vi "Main_Add User.vi"(8 "error in (no error)":errorcluster caption="에러 입력(에러 없음)") -> (0 "error out":errorcluster caption="에러 출력")   [LabVIEW 2019]
uses:
  <vilib>/Utility/config.llb/Read Key (String).vi
  <vilib>/Utility/config.llb/Read Key (U32).vi
  <vilib>/Utility/config.llb/Write Key (String).vi
  <vilib>/Utility/config.llb/Write Key (I32).vi
  <vilib>/Utility/config.llb/NI_LVConfig.lvlib
panel:
  out "권한":u32[](array[numeric])
  out "PW 2":string[](array[string])
  out "ID 2":string[](array[string])
  out "추가된 배열":string[][](array[string])
  in  "exit":bool
  in  "리스트":i32[](listbox) caption="User List"
  in  "제거 버튼":bool
  in  "추가 버튼":bool
  in  "PW":string="품명"
  in  "열거형":enum16{"Administrator", "Operator"}(ring) caption="User Authority"
  in  "ID":string="품명"
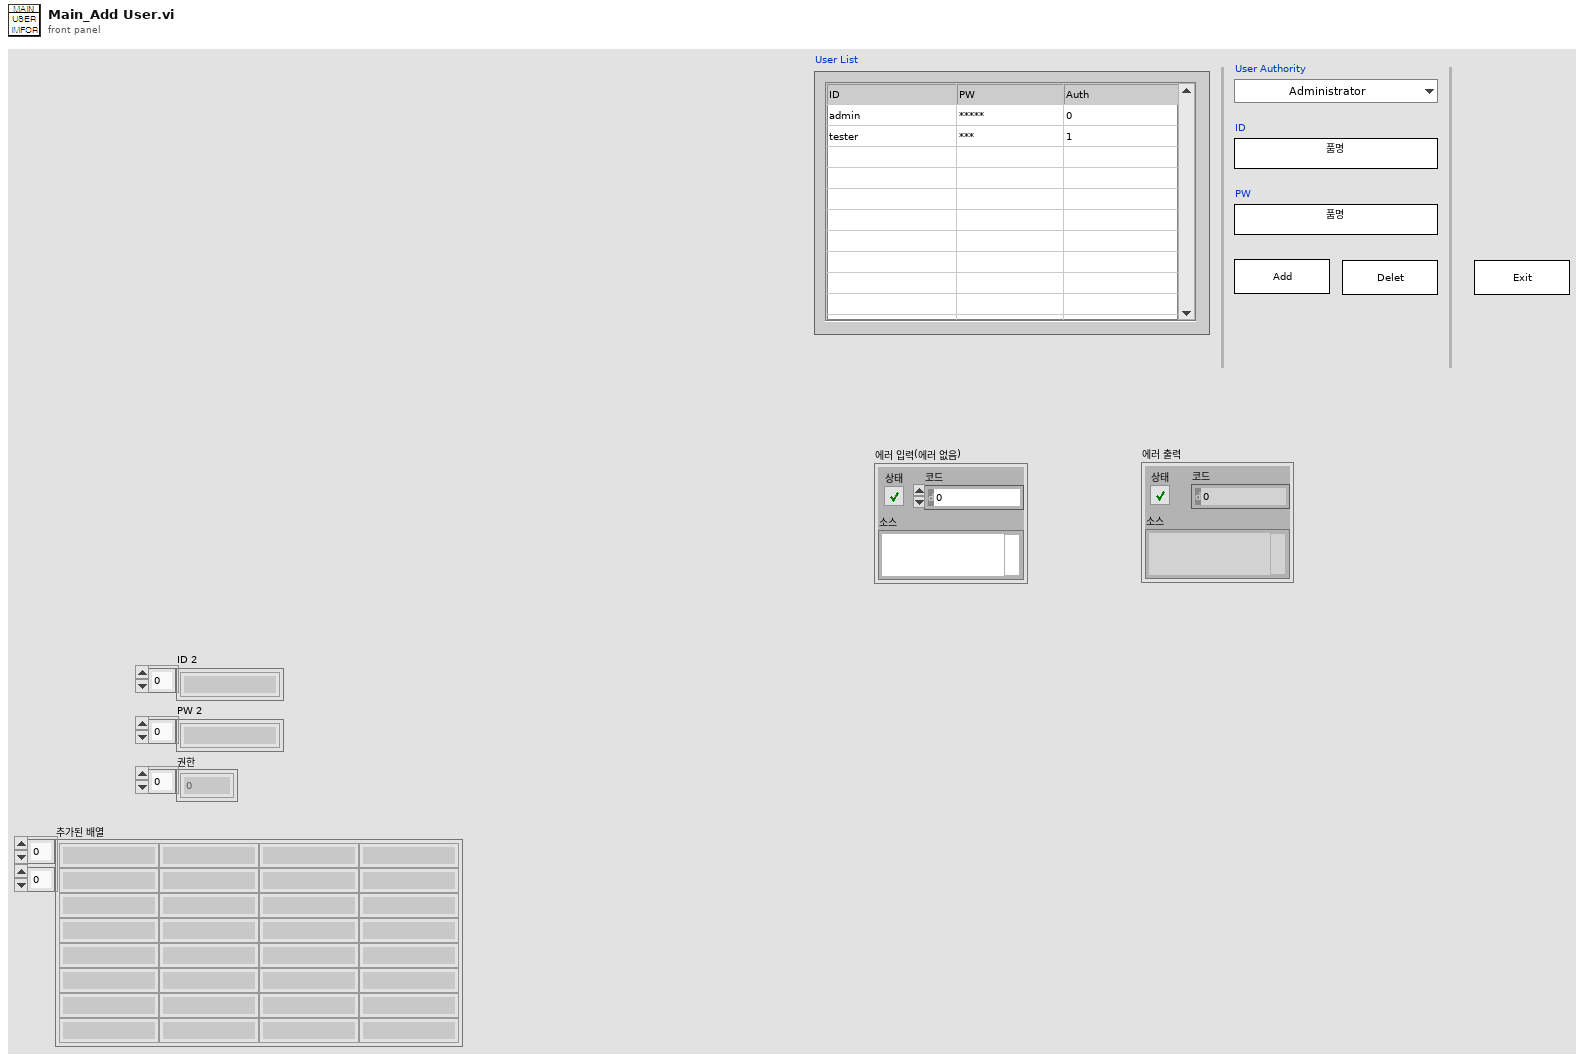
[diagram p1: front panel]
types:
  T1 = typedef "NI_LVConfig.lvlib/Config Data RefNum.ctl" = refnum<k1>
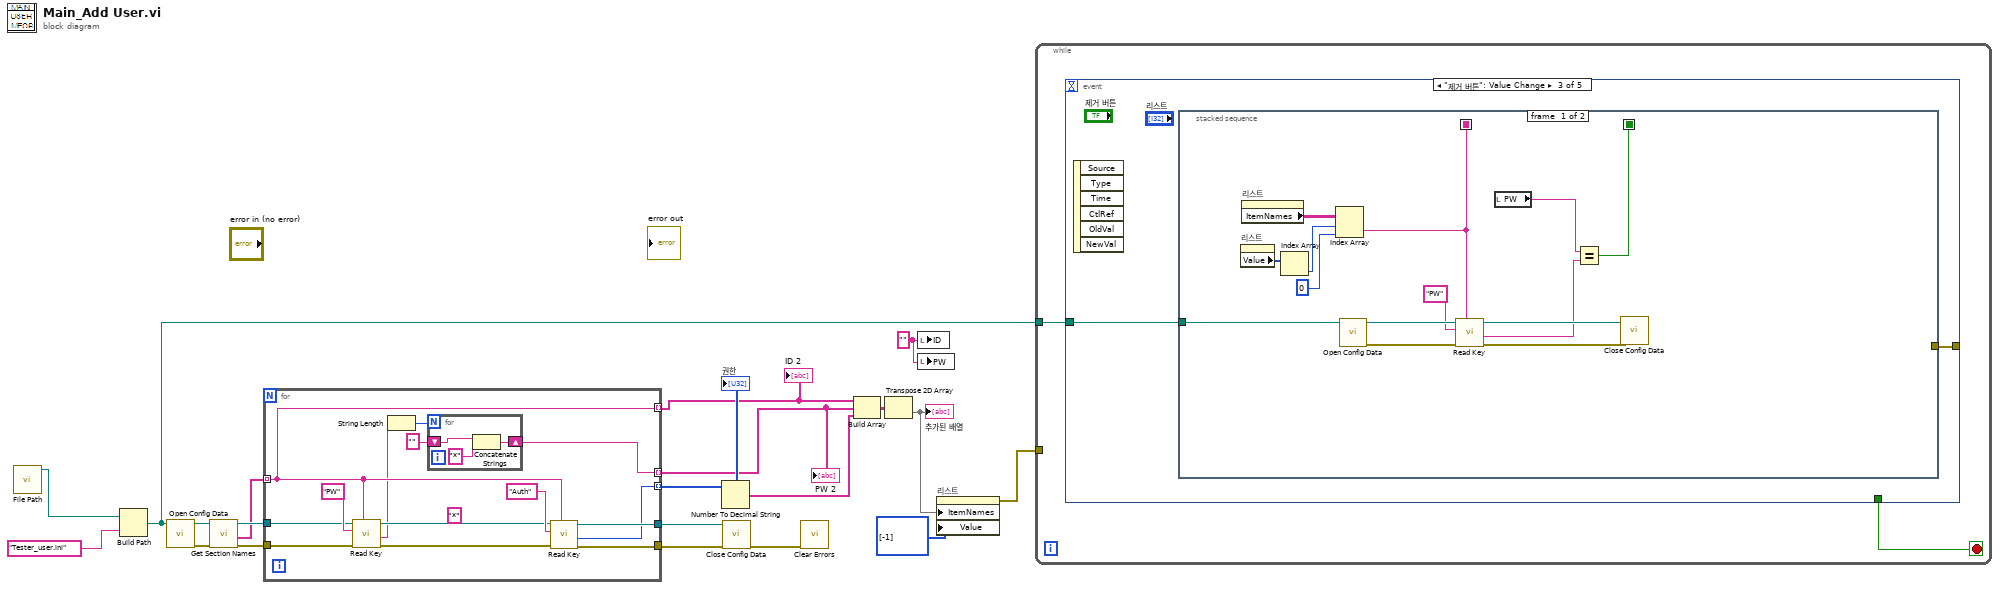
[diagram p0: block diagram]
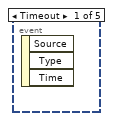
[diagram p2: hidden frame]
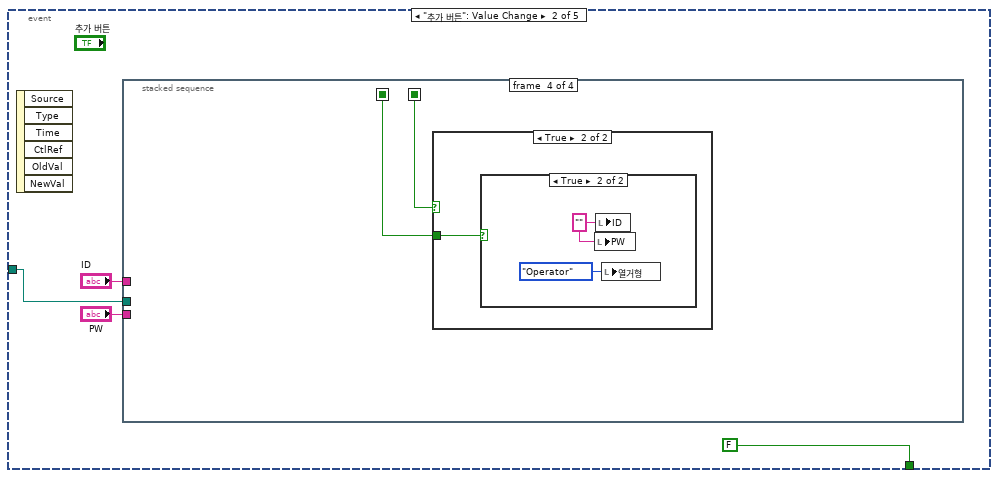
[diagram p3: hidden frame]
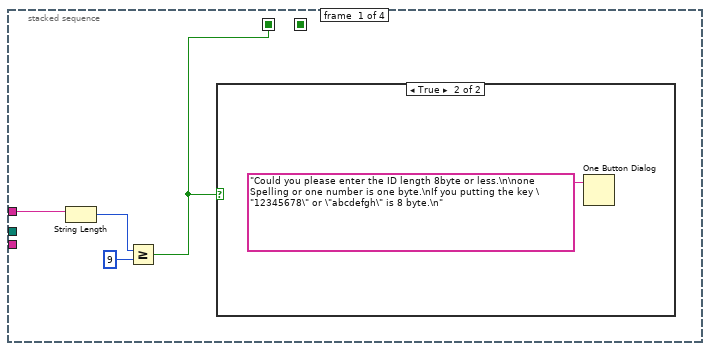
[diagram p4: hidden frame]
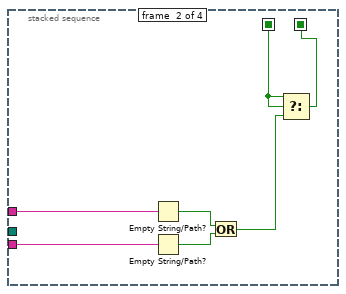
[diagram p6: hidden frame]
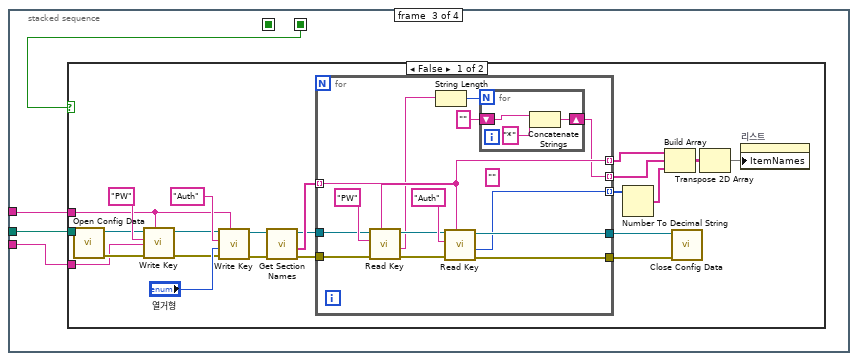
[diagram p7: hidden frame]
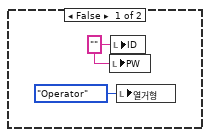
[diagram p9: hidden frame]
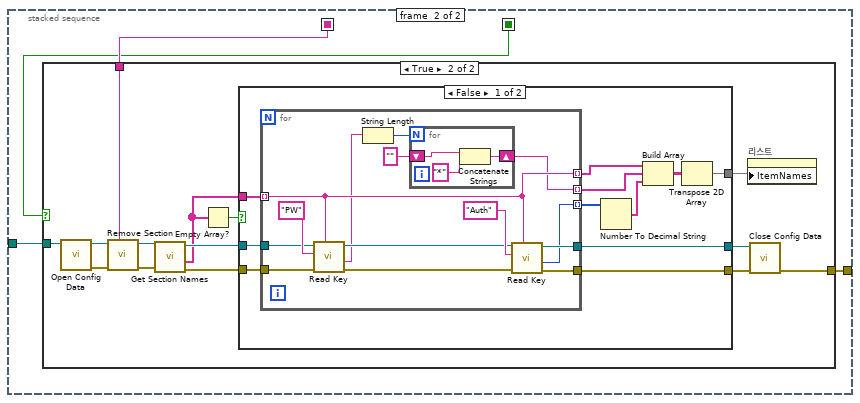
[diagram p11: hidden frame]
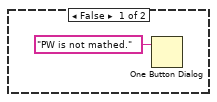
[diagram p12: hidden frame]
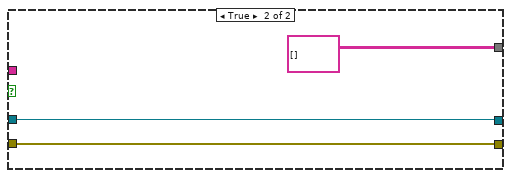
[diagram p13: hidden frame]
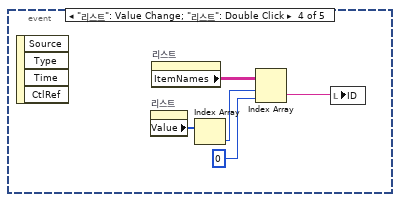
[diagram p14: hidden frame]
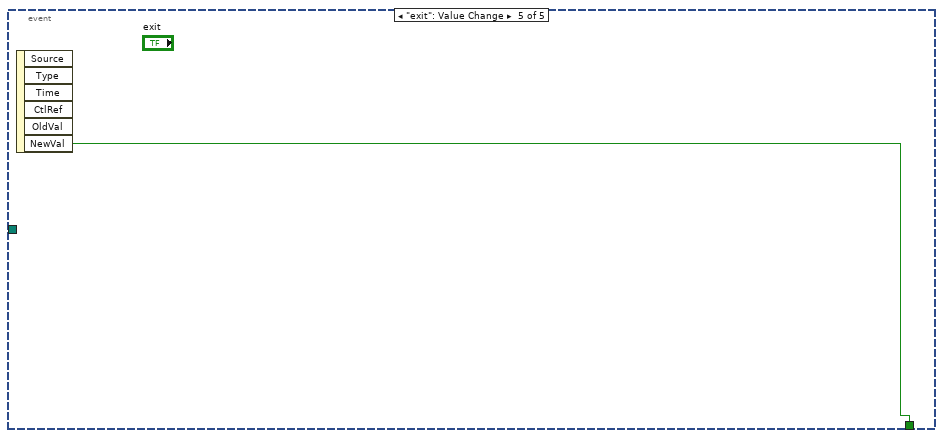
[diagram p15: hidden frame]
diagram:
  w4 = "" ("ID")
  n1 = call "File Path.vi"() -> ("condition"=w1:path)  [unwired: 7 in, 4 out]
  n2 = Build Path(base path=w1, name or relative path="Tester_user.ini" ("이름 또는 상대 경로")) -> (appended path=w6:path)
  n3 = call <vilib>:"Open Config Data.vi"("configuration file path"=w6) -> ("error out"=w15:errorcluster, "refnum"=w17:T1)  [unwired: 8 in, 1 out]
  n4 = call <vilib>:"Get Section Names.vi"("error in (no error)"=w15, "refnum"=w17) -> ("error out"=w14:errorcluster, "section names"=w13:string[], "refnum out"=w16:T1)  [unwired: 7 in]
  n5 = for {
    tunnel: [w34] -> w19
    tunnel: [w33] -> w18
    tunnel: w16 -> [w28]
    tunnel: w14 -> [w27]
    tunnel: w13 -> [w26] mode=indexing
    tunnel: [w26] -> w11 mode=indexing
    tunnel: [w22] -> w10 mode=indexing
    tunnel: [w25] -> w12 mode=indexing
    (unwired) "*"
    n6 = call-poly <vilib>:"Read Key.vi"("section"=w26, "error in (no error)"=w27, "key"="PW", "refnum"=w28) -> ("error out"=w30:errorcluster, "value"=w24:string, "refnum out"=w29:T1)  [unwired: 4 in, 1 out]
    n7 = String Length(string=w24) -> (length=w23:i32)
    n8 = for {
      N: w23 -> [_]
      shift-right: [w36] -> w22
      shift-left: "" -> [w35]
      n9 = Concatenate Strings(w35, "*") -> (w36:string)
    }
    n10 = call-poly <vilib>:"Read Key.vi"("section"=w26, "error in (no error)"=w30, "key"="Auth" ("default value"), "refnum"=w29) -> ("error out"=w34:errorcluster, "value"=w25:u32, "refnum out"=w33:T1)  [unwired: 4 in, 1 out]
  }
  "ID 2" <- w11
  "PW 2" <- w10
  "권한" <- w12
  n11 = Number To Decimal String(number=w12) -> (decimal integer string=w9:string[])  [unwired: 1 in]
  n12 = call <vilib>:"Close Config Data.vi"("error in (no error)"=w19, "refnum"=w18) -> ("error out"=w3:errorcluster)  [unwired: 8 in, 1 out]
  n13 = call <vilib>:"Clear Errors.vi"("error in (no error)"=w3) -> ()  [unwired: 5 in, 2 out]
  n14 = Build Array(w11, w10, w9) -> (w8:string[][])
  n15 = Transpose 2D Array(2D array=w8) -> (transposed array=w7:string[][])
  "추가된 배열" <- w7
  n16 = local write "ID"(w4) -> ()
  n17 = local write "PW"(w4) -> ()
  n18 = property on="리스트" class="MCListbox (strict)"("ItemNames"=w7, "Value"=i32[] [-1] ("리스트")) -> (error out=w5:errorcluster)  [unwired: 2 in, 1 out]
  n19 = while {
    tunnel: w6 -> [w39]
    tunnel: w5 -> [_]
    stop <- w38 stop-if-true
    n20 = event shown="[2] \"제거 버튼\": Value Change" {
      selector: _ -> [_ _ _ _ _]
      dyn-events: _ -> [_ _ _ _ _]
      timeout: _ -> [_ _ _ _ _]
      tunnel: w39 -> [_ w43 w108 _ _]
      tunnel: [_ FALSE _ _ w178] -> w38
      tunnel: [_ _ w107 _ _] -> _
      event Timeout {
        n21 = event-data() -> ()  [unwired: 1 in, 3 out]
      }
      event "추가 버튼": Value Change {
        n22 = event-data() -> ()  [unwired: 1 in, 6 out]
        n23 = stacked-sequence {
          seq-local: [_ w49 _ _] -> [_ _ w56 w101]
          seq-local: [w44 _ _ _] -> [_ w51 _ w100]
          tunnel: w43 -> [_ _ w59 _]
          tunnel: "ID" -> [w45 w53 w58 _]
          tunnel: "PW" -> [_ w52 w57 _]
          frame #0 {
            n24 = String Length(string=w45) -> (length=w47:i32)
            n25 = Greater Or Equal?(x=w47, y=9) -> (x >= y?=w44:bool)
            n26 = case shown="True" w44 {
              frame False {
              }
              frame True {
                n27 = One Button Dialog(message="Could you please enter the ID length 8byte or less.\n\none Spelling or one number is one byte.\nIf you putting the key \"12345678\" or \"abcdefgh\" is 8 byte.\n" ("메시지")) -> ()  [unwired: 1 in, 1 out]
              }
            }
          }
          frame #1 {
            n28 = Empty String/Path?(string/path=w53) -> (empty?=w55:bool)
            n29 = Empty String/Path?(string/path=w52) -> (empty?=w54:bool)
            n30 = Or(x=w55, y=w54) -> (x .or. y?=w50:bool)
            n31 = Select(t=w51, s=w51, f=w50) -> (s? t:f=w49:bool)
          }
          frame #2 {
            n32 = case shown="False" w56 {
              tunnel: w59 -> [w75 _]
              tunnel: w58 -> [w61 _]
              tunnel: w57 -> [w60 _]
              frame False {
                n33 = call <vilib>:"Open Config Data.vi"("configuration file path"=w75) -> ("error out"=w77:errorcluster, "refnum"=w76:T1)  [unwired: 8 in, 1 out]
                n34 = call-poly <vilib>:"Write Key.vi"("section"=w61, "error in (no error)"=w77, "value"=w60, "key"="PW", "refnum"=w76) -> ("error out"=w79:errorcluster, "refnum out"=w78:T1)  [unwired: 4 in, 1 out]
                n35 = call-poly <vilib>:"Write Key.vi"("section"=w61, "error in (no error)"=w79, "value"="열거형", "key"="Auth" ("default value"), "refnum"=w78) -> ("error out"=w62:errorcluster, "refnum out"=w63:T1)  [unwired: 4 in, 1 out]
                n36 = call <vilib>:"Get Section Names.vi"("error in (no error)"=w62, "refnum"=w63) -> ("error out"=w68:errorcluster, "section names"=w69:string[], "refnum out"=w67:T1)  [unwired: 7 in]
                n37 = for {
                  tunnel: [w96] -> w65
                  tunnel: [w95] -> w66
                  tunnel: w67 -> [w90]
                  tunnel: w68 -> [w89]
                  tunnel: w69 -> [w87] mode=indexing
                  tunnel: [w87] -> w71 mode=indexing
                  tunnel: [w83] -> w72 mode=indexing
                  tunnel: [w88] -> w70 mode=indexing
                  (unwired) "" ("value")
                  n38 = call-poly <vilib>:"Read Key.vi"("section"=w87, "error in (no error)"=w89, "key"="PW", "refnum"=w90) -> ("error out"=w92:errorcluster, "value"=w84:string, "refnum out"=w91:T1)  [unwired: 4 in, 1 out]
                  n39 = String Length(string=w84) -> (length=w86:i32)
                  n40 = call-poly <vilib>:"Read Key.vi"("section"=w87, "error in (no error)"=w92, "key"="Auth" ("default value"), "refnum"=w91) -> ("error out"=w96:errorcluster, "value"=w88:u32, "refnum out"=w95:T1)  [unwired: 4 in, 1 out]
                  n41 = for {
                    N: w86 -> [_]
                    shift-right: [w98] -> w83
                    shift-left: "" -> [w97]
                    n42 = Concatenate Strings(w97, "*") -> (w98:string)
                  }
                }
                n43 = Number To Decimal String(number=w70) -> (decimal integer string=w73:string[])  [unwired: 1 in]
                n44 = Build Array(w71, w72, w73) -> (w74:string[][])
                n45 = call <vilib>:"Close Config Data.vi"("error in (no error)"=w65, "refnum"=w66) -> ()  [unwired: 8 in, 2 out]
                n46 = Transpose 2D Array(2D array=w74) -> (transposed array=w64:string[][])
                n47 = property on="리스트" class="MCListbox (strict)"("ItemNames"=w64) -> ()  [unwired: 2 in, 2 out]
              }
              frame True {
              }
            }
          }
          frame #3 {
            n48 = case shown="True" w101 {
              tunnel: w100 -> [_ w104]
              frame False {
                w103 = "" ("ID")
                n49 = local write "PW"(w103) -> ()
                n50 = local write "ID"(w103) -> ()
                n51 = local write "열거형"(enum16{"Administrator", "Operator"}."Operator" ("열거형")) -> ()
              }
              frame True {
                n52 = case shown="True" w104 {
                  frame False {
                  }
                  frame True {
                    w105 = "" ("ID")
                    n53 = local write "PW"(w105) -> ()
                    n54 = local write "ID"(w105) -> ()
                    n55 = local write "열거형"(enum16{"Administrator", "Operator"}."Operator" ("열거형")) -> ()
                  }
                }
              }
            }
          }
        }
      }
      event "제거 버튼": Value Change {
        n56 = event-data() -> ()  [unwired: 1 in, 6 out]
        n57 = stacked-sequence {
          seq-local: [w113 _] -> [_ w124]
          seq-local: [w109 _] -> [_ w123]
          tunnel: w108 -> [w112 w126]
          tunnel: [_ w125] -> w107
          frame #0 {
            n58 = property on="리스트" class="MCListbox (strict)"() -> ("Value"=w121:i32[])  [unwired: 2 in, 2 out]
            n59 = property on="리스트" class="MCListbox (strict)"() -> ("ItemNames"=w122:string[][])  [unwired: 2 in, 2 out]
            n60 = Index Array(array=w121) -> (element=w120:i32)  [unwired: 1 in]
            n61 = Index Array(array=w122, index (row)=w120, index (col)=0 ("비활성화된 인덱스 (행)")) -> (element=w113:string)
            n62 = call <vilib>:"Open Config Data.vi"("configuration file path"=w112) -> ("error out"=w116:errorcluster, "refnum"=w115:T1)  [unwired: 8 in, 1 out]
            n63 = call-poly <vilib>:"Read Key.vi"("section"=w113, "error in (no error)"=w116, "key"="PW", "refnum"=w115) -> ("error out"=w118:errorcluster, "value"=w110:string, "refnum out"=w117:T1)  [unwired: 4 in, 1 out]
            n64 = local read "PW"() -> (w111:string)
            n65 = Equal?(x=w111, y=w110) -> (x = y?=w109:bool)
            n66 = call <vilib>:"Close Config Data.vi"("error in (no error)"=w118, "refnum"=w117) -> ()  [unwired: 8 in, 2 out]
          }
          frame #1 {
            n67 = case shown="True" w123 {
              tunnel: w126 -> [_ w139]
              tunnel: [_ w132] -> w125
              tunnel: w124 -> [_ w128]
              frame False {
                n68 = One Button Dialog(message="PW is not mathed." ("메시지")) -> ()  [unwired: 1 in, 1 out]
              }
              frame True {
                n69 = call <vilib>:"Open Config Data.vi"("configuration file path"=w139) -> ("error out"=w141:errorcluster, "refnum"=w140:T1)  [unwired: 8 in, 1 out]
                n70 = call <vilib>:"Remove Section.vi"("section"=w128, "error in (no error)"=w141, "refnum"=w140) -> ("error out"=w133:errorcluster, "refnum out"=w134:T1)  [unwired: 6 in, 1 out]
                n71 = call <vilib>:"Get Section Names.vi"("error in (no error)"=w133, "refnum"=w134) -> ("error out"=w138:errorcluster, "section names"=w131:string[], "refnum out"=w137:T1)  [unwired: 7 in]
                n72 = Empty Array?(array=w131) -> (empty?=w130:bool)
                n73 = case shown="False" w130 {
                  tunnel: w138 -> [w147 w171]
                  tunnel: w137 -> [w146 w172]
                  tunnel: [w145 w172] -> w136
                  tunnel: [w144 w171] -> w135
                  tunnel: w131 -> [w143 _]
                  tunnel: [w142 string[][] []] -> w129
                  frame False {
                    n74 = for {
                      tunnel: [w166] -> w144
                      tunnel: [w165] -> w145
                      tunnel: w146 -> [w160]
                      tunnel: w147 -> [w159]
                      tunnel: w143 -> [w158] mode=indexing
                      tunnel: [w158] -> w149 mode=indexing
                      tunnel: [w153] -> w150 mode=indexing
                      tunnel: [w157] -> w148 mode=indexing
                      n75 = call-poly <vilib>:"Read Key.vi"("section"=w158, "error in (no error)"=w159, "key"="PW", "refnum"=w160) -> ("error out"=w162:errorcluster, "value"=w154:string, "refnum out"=w161:T1)  [unwired: 4 in, 1 out]
                      n76 = String Length(string=w154) -> (length=w156:i32)
                      n77 = for {
                        N: w156 -> [_]
                        shift-right: [w168] -> w153
                        shift-left: "" -> [w167]
                        n78 = Concatenate Strings(w167, "*") -> (w168:string)
                      }
                      n79 = call-poly <vilib>:"Read Key.vi"("section"=w158, "error in (no error)"=w162, "key"="Auth" ("default value"), "refnum"=w161) -> ("error out"=w166:errorcluster, "value"=w157:u32, "refnum out"=w165:T1)  [unwired: 4 in, 1 out]
                    }
                    n80 = Number To Decimal String(number=w148) -> (decimal integer string=w151:string[])  [unwired: 1 in]
                    n81 = Build Array(w149, w150, w151) -> (w152:string[][])
                    n82 = Transpose 2D Array(2D array=w152) -> (transposed array=w142:string[][])
                  }
                  frame True {
                  }
                }
                n83 = property on="리스트" class="MCListbox (strict)"("ItemNames"=w129) -> ()  [unwired: 2 in, 2 out]
                n84 = call <vilib>:"Close Config Data.vi"("error in (no error)"=w135, "refnum"=w136) -> ("error out"=w132:errorcluster)  [unwired: 8 in, 1 out]
              }
            }
          }
        }
      }
      event "리스트": Value Change; "리스트": Double Click {
        n85 = event-data() -> ()  [unwired: 1 in, 4 out]
        n86 = property on="리스트" class="MCListbox (strict)"() -> ("Value"=w176:i32[])  [unwired: 2 in, 2 out]
        n87 = property on="리스트" class="MCListbox (strict)"() -> ("ItemNames"=w177:string[][])  [unwired: 2 in, 2 out]
        n88 = Index Array(array=w176) -> (element=w175:i32)  [unwired: 1 in]
        n89 = Index Array(array=w177, index (row)=w175, index (col)=0 ("비활성화된 인덱스 (행)")) -> (element=w173:string)
        n90 = local write "ID"(w173) -> ()
      }
      event "exit": Value Change {
        n91 = event-data() -> ("NewVal"=w178:bool)  [unwired: 1 in, 5 out]
      }
    }
  }
